vi "Make JSON Array.vi"(6 "Pretty Print?":bool, 8 "error in (no error)":errorcluster, 9 "JSON Elements":string[](array[string])) -> (0 "error out":errorcluster, 3 "<JSON>":string caption="<JSON>Array")   [LabVIEW 2021, in "json.facade.lvlib"]
doc: "Format a JSON Array out of an array of JSON items."
uses:
  json.facade.lvlib
  jsontext/JSONtext.lvlib
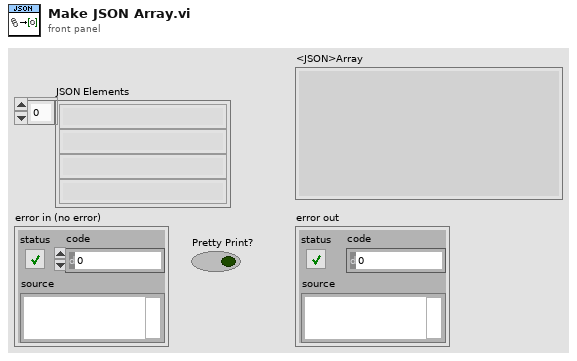
[diagram p1: front panel]
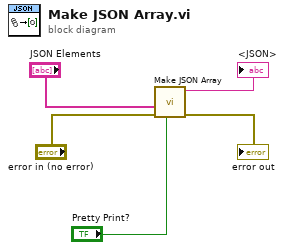
[diagram p0: block diagram]
diagram:
  n1 = call "Make JSON Array.vi"("Pretty Print?"="Pretty Print?", "error in (no error)"="error in (no error)", "JSON Elements"="JSON Elements") -> ("error out"=→"error out":errorcluster, "<JSON>"=→"<JSON>":string)  [unwired: 7 in]
